vi "Field within range.vi"(0 "ith step":u16, 1 "RampParameter":dbl[](array[numeric])=[0.0, 30.0, 1.0, 20.0] format="%.2f", 3 "Maximum Allowed Current":dbl=100.0 format="%.2f", 4 "stopCycle":bool) -> (5 "Output String":string, 6 "Ramp Speed":dbl=20.0 format="%.2f", 7 "Continue?":bool=TRUE)   [LabVIEW 2019]
doc: "This Vi extract current field and set the scan continue boolean variable.\n\nThe field step can be either positive or negative.\n\nIf any of the absolute field value exceeds the maximum allowed limit, it will be replaced with the maximum field value itself"
panel:
  out "Field Array List":dbl[](array[numeric])=[0.0, 0.5, 1.0, 1.5, 2.0, 2.5, 3.0, 3.5, 4.0, 4.5, 5.0, 5.5, 6.0, 6.5, 7.0, 7.5, 8.0, 8.5, 9.0, 9.5, 10.0, 10.5, 11.0, 11.5, 12.0, 12.5, 13.0, 13.5, 14.0, 14.5, 15.0, 15.5, 16.0, 16.5, 17.0, 17.5, 18.0, 18.5, 19.0, 19.5, 20.0, 20.5, 21.0, 21.5, 22.0, 22.5, 23.0, 23.5, 24.0, 24.5, 25.0, 25.5, 26.0, 26.5, 27.0, 27.5, 28.0, 28.5, 29.0, 29.5, 30.0, 30.5, 31.0, 31.5, 32.0, 32.5, 33.0, 33.5, 34.0, 34.5, 35.0, 35.5, 36.0, 36.5, 37.0, 37.5, 38.0, 38.5, 39.0, 39.5, 40.0, 40.5, 41.0, 41.5, 42.0, 42.5, 43.0, 43.5, 44.0, 44.5]
  out "Goto Field":dbl format="%.2f"
  out "Field Step":dbl=0.5 format="%.2f"
  out "Final Field":dbl=45.0 format="%.2f"
  out "Initial Field":dbl format="%.2f"
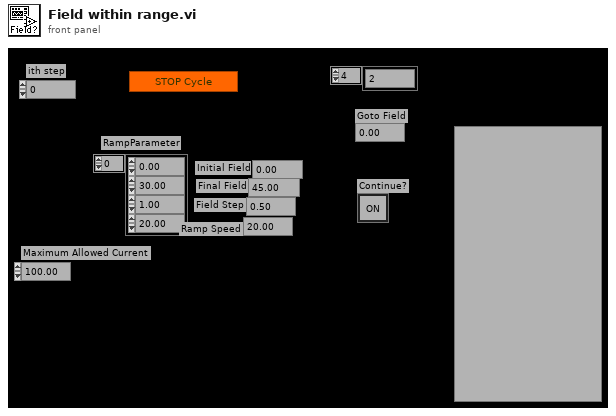
[diagram p1: front panel]
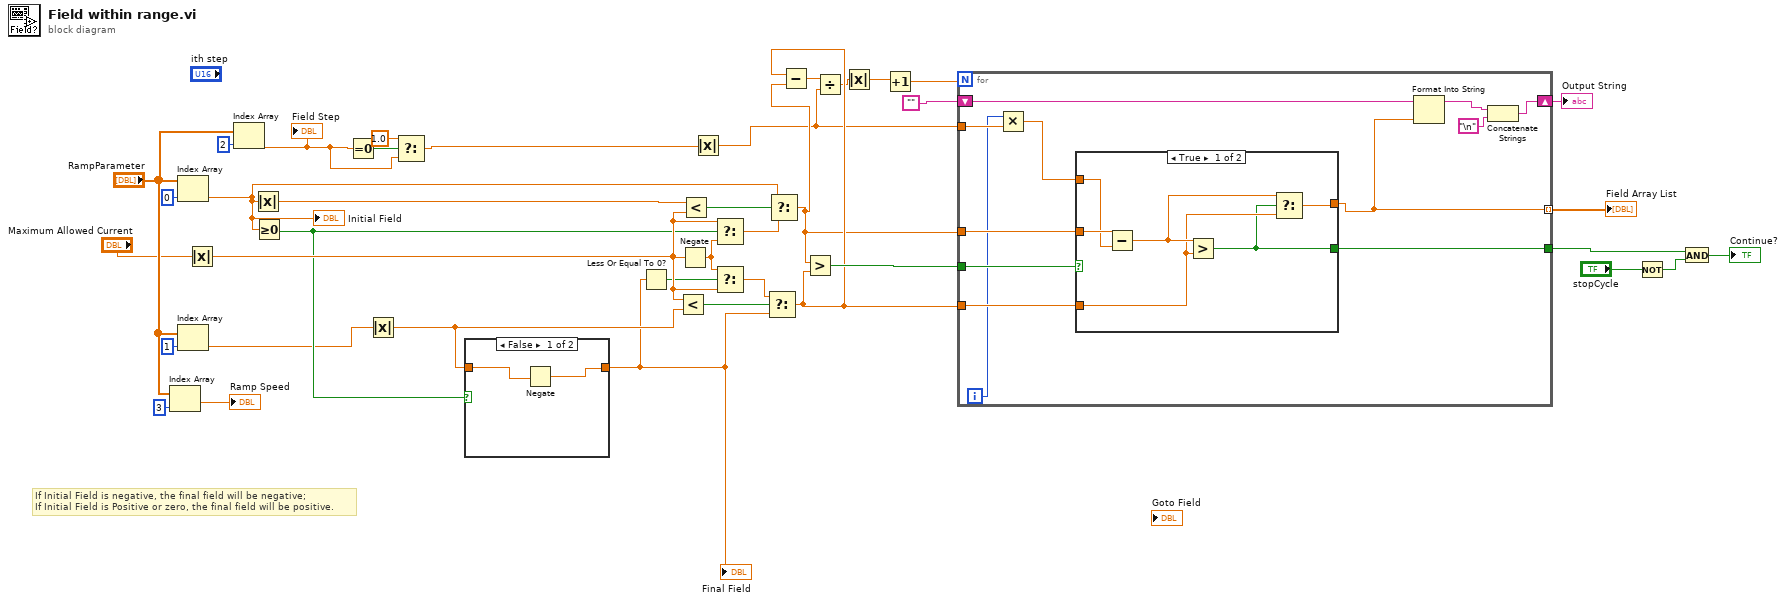
[diagram p0: block diagram]
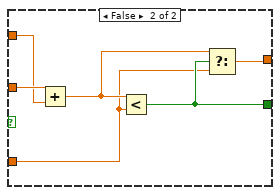
[diagram p2: hidden frame]
diagram:
  # "If Initial Field is negative, the final field will be negative;\nIf Initial Field is Positive or zero, the final field will be positive."
  n1 = Index Array(array="RampParameter", index=3) -> (element=→"Ramp Speed":dbl)
  n2 = Index Array(array="RampParameter", index=0) -> (element=w28:dbl)
  "Initial Field" <- w28
  n3 = Index Array(array="RampParameter", index=1) -> (element=w24:dbl)
  n4 = Absolute Value(x="Maximum Allowed Current") -> (abs(x)=w35:dbl)
  n5 = Index Array(array="RampParameter", index=2) -> (element=w20:dbl)
  "Field Step" <- w20
  n6 = Absolute Value(x=w28) -> (abs(x)=w36:dbl)
  n7 = Greater Or Equal To 0?(x=w28) -> (x >= 0?=w26:bool)
  n8 = Equal To 0?(x=w20) -> (x = 0?=w21:bool)
  n9 = Absolute Value(x=w24) -> (abs(x)=w25:dbl)
  n10 = Select(t=1.0, s=w21, f=w20) -> (s? t:f=w18:dbl)
  n11 = case shown="False" w26 {
    tunnel: w25 -> [w41 w42]
    tunnel: [w40 w42] -> w23
    frame False {
      n12 = Negate(x=w41) -> (-x=w40:dbl)
    }
    frame True {
    }
  }
  "Final Field" <- w23
  n13 = Less Or Equal To 0?(x=w23) -> (x <= 0?=w13:bool)
  n14 = Less?(x=w35, y=w25) -> (x < y?=w15:bool)
  n15 = Negate(x=w35) -> (-x=w12:dbl)
  n16 = Less?(x=w36, y=w35) -> (x < y?=w16:bool)
  n17 = Absolute Value(x=w18) -> (abs(x)=w7:dbl)
  n18 = Select(t=w35, s=w26, f=w12) -> (s? t:f=w14:dbl)
  n19 = Select(t=w12, s=w13, f=w35) -> (s? t:f=w11:dbl)
  n20 = Select(t=w11, s=w15, f=w23) -> (s? t:f=w10:dbl)
  n21 = Select(t=w28, s=w16, f=w14) -> (s? t:f=w9:dbl)
  n22 = Subtract(x=w10, y=w9) -> (x-y=w8:dbl)
  n23 = Greater?(x=w9, y=w10) -> (0:w17:bool)
  n24 = Divide(x=w8, y=w7) -> (x/y=w6:dbl)
  n25 = Absolute Value(x=w6) -> (abs(x)=w4:dbl)
  n26 = Increment(x=w4) -> (x+1=w3:dbl)
  n27 = for {
    N: w3 -> [_]
    tunnel: [w54] -> w34
    tunnel: w17 -> [w53]
    tunnel: w7 -> [w52]
    tunnel: w9 -> [w51]
    tunnel: w10 -> [w50]
    tunnel: [w47] -> w5 mode=indexing
    shift-right: [w43] -> w2
    shift-left: "" -> [w45]
    i -> [w48]
    n28 = Multiply(x=w48, y=w52) -> (x*y=w49:dbl)
    n29 = case shown="True" w53 {
      tunnel: [w55 w63] -> w54
      tunnel: w51 -> [w60 w66]
      tunnel: w50 -> [w56 w62]
      tunnel: w49 -> [w59 w65]
      tunnel: [w58 w61] -> w47
      frame True {
        n30 = Subtract(x=w60, y=w59) -> (x-y=w57:dbl)
        n31 = Greater?(x=w57, y=w56) -> (0:w55:bool)
        n32 = Select(t=w57, s=w55, f=w56) -> (s? t:f=w58:dbl)
      }
      frame False {
        n33 = Add(x=w66, y=w65) -> (x+y=w64:dbl)
        n34 = Less?(x=w64, y=w62) -> (x < y?=w63:bool)
        n35 = Select(t=w64, s=w63, f=w62) -> (s? t:f=w61:dbl)
      }
    }
    n36 = Format Into String(initial string=w45, w47) -> (resulting string=w44:string)  [unwired: 2 in, 1 out]
    n37 = Concatenate Strings(w44, "\n") -> (w43:string)
  }
  "Field Array List" <- w5
  "Output String" <- w2
  n38 = Not(x="stopCycle") -> (.not. x?=w39:bool)
  n39 = And(x=w34, y=w39) -> (x .and. y?=→"Continue?":bool)
